vi "Send ReadData.vi"(7 "Message Priority (Normal)":T1=enum."Normal", 8 "error in (no error)":errorcluster, 10 "LogicName":string, 11 "Message Enqueuer":refnum<class "Message Enqueuer.lvclass">) -> (0 "error out":errorcluster, 2 "Data":variant, 3 "Message Enqueuer out":refnum<class "Message Enqueuer.lvclass">)   [LabVIEW 2025, in "PLC_Module.lvlib" / "ReadData Msg.lvclass"]
doc: "This VI sends the message to an actor."
uses:
  ReadData Msg.lvclass
  <vilib>/ActorFramework/Message Enqueuer/Message Enqueuer.lvclass
  <vilib>/ActorFramework/Message Enqueuer/Message Priority.ctl
  C:/Program Files (x86)/National Instruments/LabVIEW 2025/vi.lib/ActorFramework/Message/Message.lvclass
  ReadData Msg.lvclass/ReadData Msg.ctl
  <vilib>/ActorFramework/Message Enqueuer/Message Enqueuer.lvclass/Message Enqueuer.ctl
  <vilib>/ActorFramework/Message Priority Queue/Priority Enqueue.vi
  D:/Hardware/PLC/PLC_Module/PLC_Module Messages/ReadData Msg/ReadData Msg.lvclass
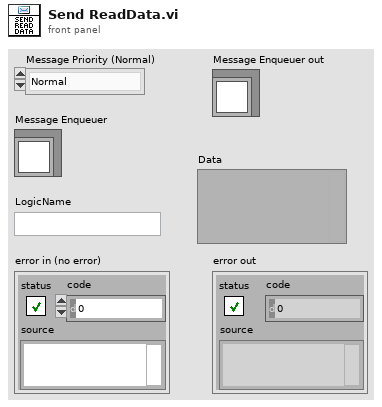
[diagram p1: front panel]
types:
  T1 = typedef "Actor Framework.lvlib/Message Enqueuer.lvclass/Message Priority.ctl" = enum16{"Low", "Normal", "High"}
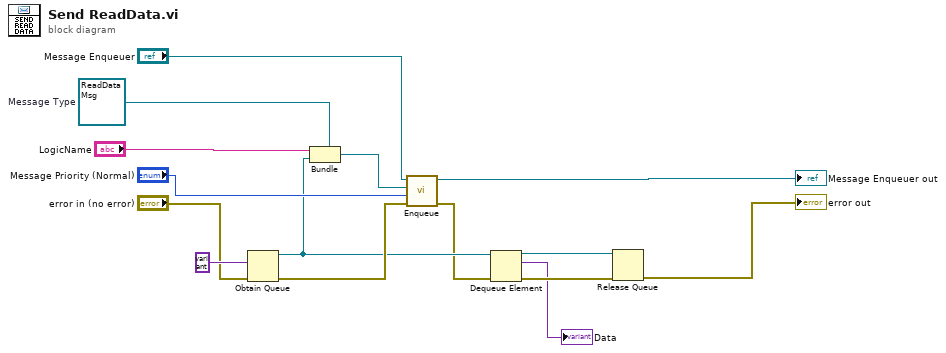
[diagram p0: block diagram]
diagram:
  w14 = refnum<class "ReadData Msg.lvclass"> refnum  # Message Type
  n1 = Obtain Queue(element data type=variant, error in (no error)="error in (no error)") -> (queue out=w6:refnum<queue>, error out=w7:errorcluster)  [unwired: 3 in, 1 out]
  n2 = Bundle(cluster=w14, "LogicName", w6) -> (w13:refnum<class "ReadData Msg.lvclass">)
  n3 = call <vilib>:"Enqueue.vi"("error in (no error)"=w7, "Message Priority (Normal)"="Message Priority (Normal)", "Message"=w13, "Message Enqueuer in"="Message Enqueuer") -> ("error out"=w5:errorcluster, "Message Enqueuer out"=→"Message Enqueuer out":refnum<class "Message Enqueuer.lvclass">)  [unwired: 6 in]
  n4 = Dequeue Element(queue=w6, error in (no error)=w5) -> (queue out=w4:refnum<queue>, element=→"Data":variant, error out=w3:errorcluster)  [unwired: 1 in, 1 out]
  n5 = Release Queue(queue=w4, error in (no error)=w3) -> (error out=→"error out":errorcluster)  [unwired: 1 in, 2 out]
